vi "Top level_ Node FTP and STAT software.vi"() -> ()   [LabVIEW 2010]
uses:
  <vilib>/Utility/config.llb/NI_LVConfig.lvlib
  <vilib>/Utility/sysdir.llb/System Directory Type.ctl
  <vilib>/Utility/config.llb/Write Key (Boolean).vi
  FTP Credintials.ctl
panel:
  in  "Top level Tabs":enum32{"FTP Connection & Directories", "Page 2"}(tab)
  in  "Manual FTP":bool
  in  "Manual Archive":bool
  in  "ShutDown":bool
  in  "FTP Creds":T1 {"FTP Timeout (S)" min=0 max=10 step=1}
  in  "Archive Location 2":path caption="(Optional) External Directory To Archive *.RAT files"
  in  "Archive Location":path=path "C:/Archive" caption="Directory To Archive *.RAT files"
  in  "Rats Location":path=path "C:/Incoming" caption="Directory To Find *.RAT files"
  # "DIRECTORY SETUP"
  # "FTP SETUP"
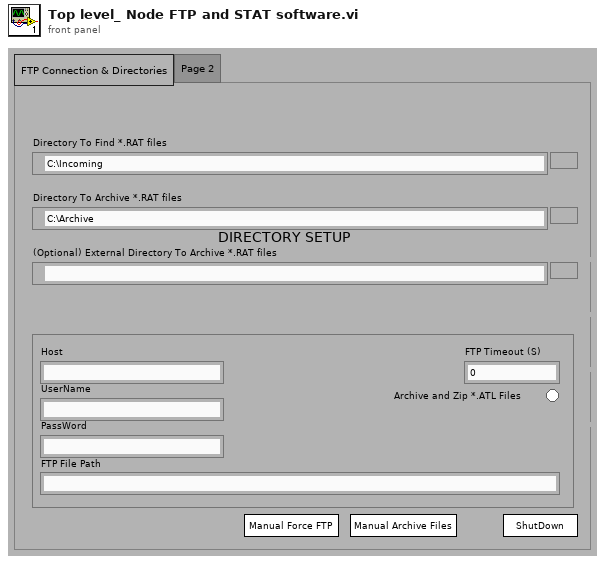
[diagram p1: front panel]
types:
  T1 = typedef "FTP Credintials.ctl" = cluster{"Host":string, "UserName":string, "PassWord":string, "FTP File Path":string, "FTP Timeout (S)":i32, "Use ATL":bool}
  T2 = typedef "System Directory Type.ctl" = i32
  T3 = cluster{"INI Section":string, "INI Key":string, "Use ATL":bool}
  T4 = cluster{"INI section (in)":string, "INI key (in)":string, "Value":string}
  T5 = typedef "NI_LVConfig.lvlib/Config Data RefNum.ctl" = refnum<k1>
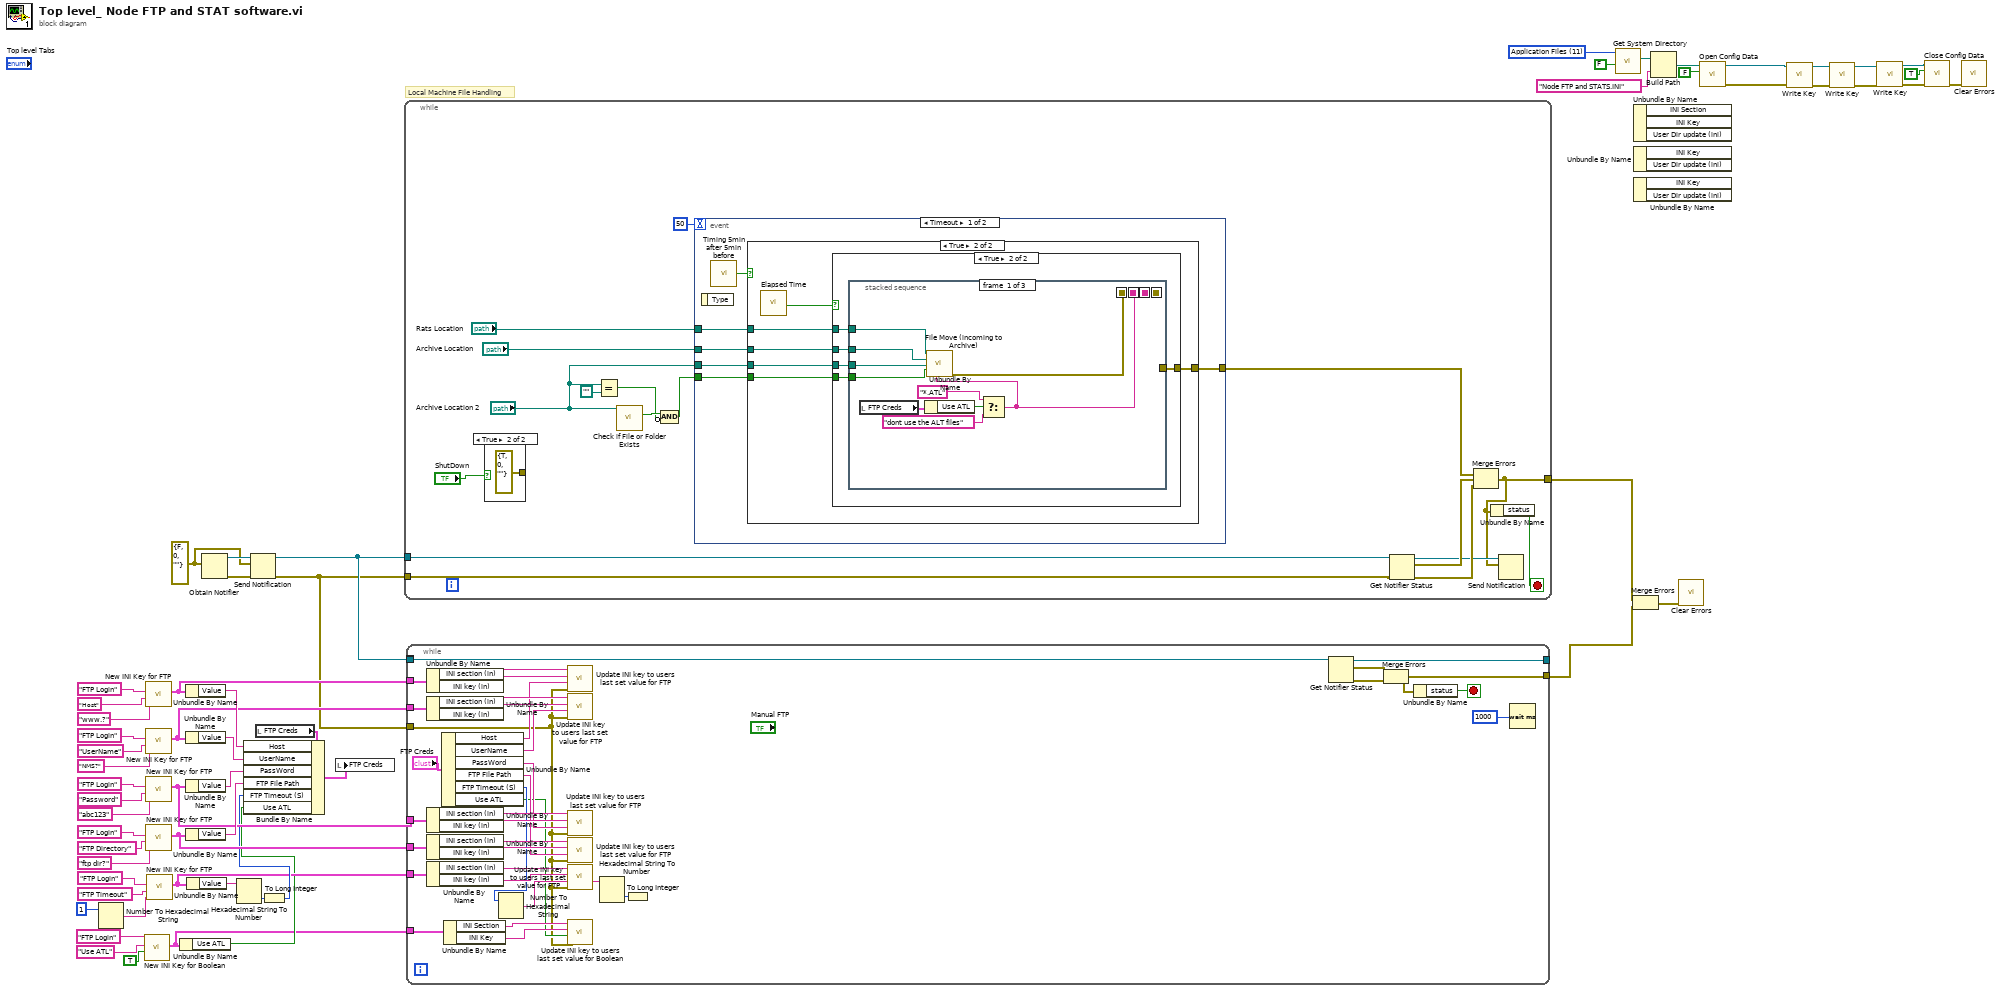
[diagram p0: block diagram]
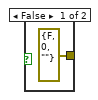
[diagram p2: hidden frame]
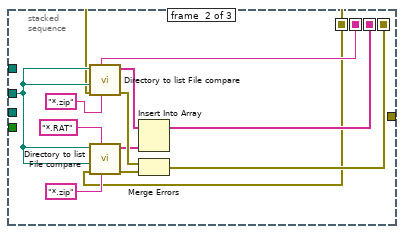
[diagram p5: hidden frame]
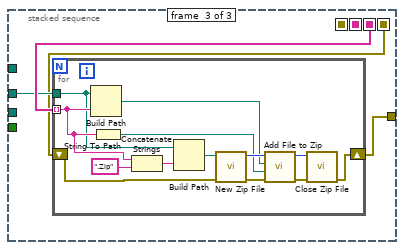
[diagram p6: hidden frame]
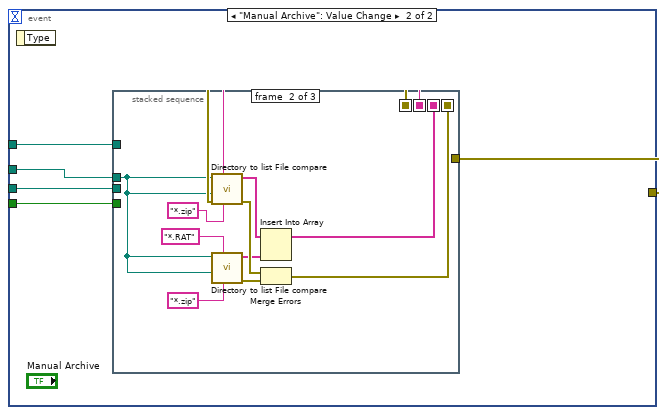
[diagram p7: hidden frame]
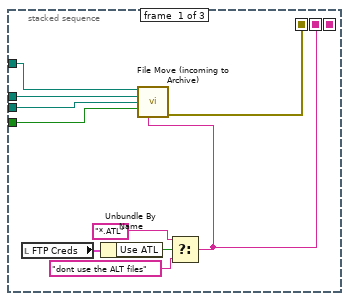
[diagram p8: hidden frame]
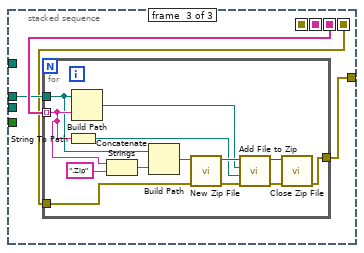
[diagram p9: hidden frame]
diagram:
  w15 = T2 11 items=["User Home"=0, "User Desktop"=1, "User Documents"=2, "User Application Data"=3, "User Preferences"=4, "User Temporary"=5, "Public Documents"=6, "Public Application Data"=7, "Public Preferences"=8, "Public Cache"=13, "System Core Libraries"=9, "System Installed Libraries"=10, "Application Files"=11, "Boot Volume Root"=12] ("system directory type")
  w23 = errorcluster {"status"=FALSE, "code"=0, "source"=""} ("error in (no error)")
  # "Local Machine File Handling"
  n1 = Number To Hexadecimal String(2:1) -> (0:w34:string)  [unwired: 1 in]
  n2 = call "New INI Key for Boolean.vi"("Use ATL"=TRUE, "INI key (in)"="Use ATL", "INI section (in)"="FTP Login") -> ("output cluster"=w25:T3)  [unwired: 8 in]
  n3 = call "New INI Key for FTP.vi"("Value"="www.?", "INI key (in)"="Host", "INI section (in)"="FTP Login") -> ("output cluster"=w43:T4)  [unwired: 7 in]
  n4 = call "New INI Key for FTP.vi"("Value"="NMS?", "INI key (in)"="UserName", "INI section (in)"="FTP Login") -> ("output cluster"=w42:T4)  [unwired: 7 in]
  n5 = call "New INI Key for FTP.vi"("Value"="abc123", "INI key (in)"="Password", "INI section (in)"="FTP Login") -> ("output cluster"=w41:T4)  [unwired: 7 in]
  n6 = call "New INI Key for FTP.vi"("Value"="ftp dir?", "INI key (in)"="FTP Directory", "INI section (in)"="FTP Login") -> ("output cluster"=w40:T4)  [unwired: 7 in]
  n7 = call "New INI Key for FTP.vi"("Value"=w34, "INI key (in)"="FTP Timeout", "INI section (in)"="FTP Login") -> ("output cluster"=w30:T4)  [unwired: 7 in]
  n8 = Unbundle By Name(w25) -> ("Use ATL"=w26:bool)
  n9 = Unbundle By Name(w43) -> ("Value"=w47:string)
  n10 = Unbundle By Name(w42) -> ("Value"=w46:string)
  n11 = Unbundle By Name(w41) -> ("Value"=w45:string)
  n12 = Unbundle By Name(w40) -> ("Value"=w44:string)
  n13 = Unbundle By Name(w30) -> ("Value"=w33:string)
  n14 = Obtain Notifier(notification data type=w23) -> (notifier out=w24:refnum<notifier>, error out=w22:errorcluster)  [unwired: 3 in, 1 out]
  n15 = Hexadecimal String To Number(string=w33) -> (number=w32:u32)  [unwired: 2 in, 1 out]
  n16 = Send Notification(notification=w23, notifier=w24, error in (no error)=w22) -> (notifier out=w21:refnum<notifier>, error out=w20:errorcluster)
  n17 = local read "FTP Creds"() -> (w38:T1)
  n18 = To Long Integer(number=w32) -> (32bit integer=w31:i32)
  n19 = Bundle By Name(cluster=w38, "Host"=w47, "UserName"=w46, "PassWord"=w45, "FTP File Path"=w44, "FTP Timeout (S)"=w31, "Use ATL"=w26) -> (w39:T1)
  n20 = local write "FTP Creds"(w39) -> ()
  n21 = while {
    tunnel: w21 -> [w71]
    tunnel: w20 -> [w69]
    tunnel: [w64] -> w19
    stop <- w67 stop-if-true
    n22 = case shown="True" "ShutDown" {
      tunnel: [errorcluster {"status"=FALSE, "code"=0, "source"=""} ("error in (no error)") errorcluster {"status"=TRUE, "code"=0, "source"=""} ("error in (no error)")] -> _
      frame False {
      }
      frame True {
      }
    }
    n23 = Equal?(x="Archive Location 2", y=path "") -> (x = y?=w74:bool)
    n24 = call <vilib>:"Check if File or Folder Exists.vi"("path"="Archive Location 2") -> ("file or folder exists?"=w75:bool)  [unwired: 8 in, 2 out]
    n25 = Compound Arithmetic op=AND(w75, invert w74) -> (w73:bool)
    n26 = event shown="[0] Timeout" {
      selector: _ -> [_ _]
      dyn-events: _ -> [_ _]
      timeout: 50 -> [_ _]
      tunnel: "Rats Location" -> [w84 w139]
      tunnel: "Archive Location" -> [w83 w138]
      tunnel: "Archive Location 2" -> [w82 w137]
      tunnel: w73 -> [w81 w136]
      tunnel: [w80 w135] -> w65
      event Timeout {
        n27 = event-data() -> ()  [unwired: 1 in, 1 out]
        n28 = call "Timing 5min after 5min before.vi"() -> ("Mid Hour"=w79:bool)  [unwired: 5 in]
        n29 = case shown="True" w79 {
          tunnel: w84 -> [_ w90]
          tunnel: w83 -> [_ w89]
          tunnel: w82 -> [_ w88]
          tunnel: w81 -> [_ w87]
          tunnel: [_ w86] -> w80
          frame False {
          }
          frame True {
            n30 = call "Elapsed Time"() -> ("Time has Elapsed"=w85:bool)  [unwired: 12 in, 7 out]
            n31 = case shown="True" w85 {
              tunnel: w90 -> [_ w95]
              tunnel: w89 -> [_ w94]
              tunnel: w88 -> [_ w93]
              tunnel: w87 -> [_ w92]
              tunnel: [_ w91] -> w86
              frame False {
              }
              frame True {
                n32 = stacked-sequence {
                  seq-local: [_ w107 _] -> [_ _ w121]
                  seq-local: [w101 _ _] -> [_ w113 _]
                  seq-local: [w100 _ _] -> [_ w106 _]
                  seq-local: [_ w110 _] -> [_ _ w119]
                  tunnel: w95 -> [w96 _ _]
                  tunnel: w94 -> [w97 w114 w120]
                  tunnel: w93 -> [w98 _ _]
                  tunnel: w92 -> [w99 _ _]
                  tunnel: [_ _ w118] -> w91
                  frame #0 {
                    n33 = local read "FTP Creds"() -> (w105:T1)
                    n34 = Unbundle By Name(w105) -> ("Use ATL"=w104:bool)
                    n35 = Select(t="*.ATL" ("pattern"), s=w104, f="dont use the ALT files" ("pattern")) -> (s? t:f=w101:string)
                    n36 = call "File Move (incoming to Archive).vi"("Rats Location"=w96, "Archive Location"=w97, "Archive Location 2"=w98, "Archive 2 valid path"=w99, "pattern"=w101) -> ("error IO"=w100:errorcluster)  [unwired: 10 in]
                  }
                  frame #1 {
                    n37 = call "Directory to list File compare.vi"("2nd File Type(s)(*.txt *.CSV)"="*.zip", "1st File Type(s)(*.txt *.CSV)"=w113, "error in (no error)"=w106, "2nd Directory (Zip)"=w114, "1st Directory (RATS)"=w114) -> ("error out"=w112:errorcluster, "Unmanaged Files"=w109:string[])  [unwired: 4 in, 1 out]
                    n38 = call "Directory to list File compare.vi"("2nd File Type(s)(*.txt *.CSV)"="*.zip", "1st File Type(s)(*.txt *.CSV)"="*.RAT" ("2nd File Type(s)(*.txt *.CSV)"), "error in (no error)"=w106, "2nd Directory (Zip)"=w114, "1st Directory (RATS)"=w114) -> ("error out"=w111:errorcluster, "Unmanaged Files"=w108:string[])  [unwired: 4 in, 1 out]
                    n39 = Insert Into Array(array=w109, new element=w108) -> (w107:string[])  [unwired: 1 in]
                    n40 = Merge Errors(w112, w111) -> (w110:errorcluster)
                  }
                  frame #2 {
                    n41 = for {
                      tunnel: w121 -> [w123] mode=indexing
                      tunnel: w120 -> [w122]
                      shift-right: [w128] -> w118
                      shift-left: w119 -> [w129]
                      n42 = Build Path(base path=w122, name or relative path=w123) -> (appended path=w126:path)
                      n43 = String To Path(string=w123) -> (path=w130:path)
                      n44 = Concatenate Strings(w123, ".Zip" ("name or relative path")) -> (w124:string)
                      n45 = Build Path(base path=w122, name or relative path=w124) -> (appended path=w127:path)
                      n46 = call <vilib>:"New Zip File.vi"("error in (no error)"=w129, "target"=w127) -> ("error out"=w131:errorcluster, "zip file out"=w134:i64)  [unwired: 3 in, 1 out]
                      n47 = call <vilib>:"Add File to Zip.vi"("error in (no error)"=w131, "destination path in zip"=w130, "source file path"=w126, "zip file in"=w134) -> ("error out"=w133:errorcluster, "zip file out"=w132:i64)  [unwired: 6 in]
                      n48 = call <vilib>:"Close Zip File.vi"("error in (no error)"=w133, "zip file in"=w132) -> ("error out"=w128:errorcluster)  [unwired: 5 in]
                    }
                  }
                }
              }
            }
          }
        }
      }
      event "Manual Archive": Value Change {
        n49 = event-data() -> ()  [unwired: 1 in, 1 out]
        n50 = stacked-sequence {
          seq-local: [_ w150 _] -> [_ _ w165]
          seq-local: [w141 _ _] -> [_ w156 _]
          seq-local: [w140 _ _] -> [_ w160 _]
          seq-local: [_ w153 _] -> [_ _ w163]
          tunnel: w139 -> [w142 _ _]
          tunnel: w138 -> [w143 w157 w164]
          tunnel: w137 -> [w144 _ _]
          tunnel: w136 -> [w145 _ _]
          tunnel: [_ _ w162] -> w135
          frame #0 {
            n51 = local read "FTP Creds"() -> (w149:T1)
            n52 = Unbundle By Name(w149) -> ("Use ATL"=w148:bool)
            n53 = Select(t="*.ATL" ("pattern"), s=w148, f="dont use the ALT files" ("pattern")) -> (s? t:f=w141:string)
            n54 = call "File Move (incoming to Archive).vi"("Rats Location"=w142, "Archive Location"=w143, "Archive Location 2"=w144, "Archive 2 valid path"=w145, "pattern"=w141) -> ("error IO"=w140:errorcluster)  [unwired: 10 in]
          }
          frame #1 {
            n55 = call "Directory to list File compare.vi"("2nd File Type(s)(*.txt *.CSV)"="*.zip", "1st File Type(s)(*.txt *.CSV)"=w156, "error in (no error)"=w160, "2nd Directory (Zip)"=w157, "1st Directory (RATS)"=w157) -> ("error out"=w155:errorcluster, "Unmanaged Files"=w152:string[])  [unwired: 4 in, 1 out]
            n56 = call "Directory to list File compare.vi"("2nd File Type(s)(*.txt *.CSV)"="*.zip", "1st File Type(s)(*.txt *.CSV)"="*.RAT" ("2nd File Type(s)(*.txt *.CSV)"), "2nd Directory (Zip)"=w157, "1st Directory (RATS)"=w157) -> ("error out"=w154:errorcluster, "Unmanaged Files"=w151:string[])  [unwired: 5 in, 1 out]
            n57 = Insert Into Array(array=w152, new element=w151) -> (w150:string[])  [unwired: 1 in]
            n58 = Merge Errors(w155, w154) -> (w153:errorcluster)
          }
          frame #2 {
            n59 = for {
              tunnel: w165 -> [w167] mode=indexing
              tunnel: w164 -> [w166]
              tunnel: w163 -> [w173]
              tunnel: [w172] -> w162
              n60 = String To Path(string=w167) -> (path=w174:path)
              n61 = Build Path(base path=w166, name or relative path=w167) -> (appended path=w170:path)
              n62 = Concatenate Strings(w167, ".Zip" ("name or relative path")) -> (w168:string)
              n63 = Build Path(base path=w166, name or relative path=w168) -> (appended path=w171:path)
              n64 = call <vilib>:"New Zip File.vi"("error in (no error)"=w173, "target"=w171) -> ("error out"=w175:errorcluster, "zip file out"=w178:i64)  [unwired: 3 in, 1 out]
              n65 = call <vilib>:"Add File to Zip.vi"("error in (no error)"=w175, "destination path in zip"=w174, "source file path"=w170, "zip file in"=w178) -> ("error out"=w177:errorcluster, "zip file out"=w176:i64)  [unwired: 6 in]
              n66 = call <vilib>:"Close Zip File.vi"("error in (no error)"=w177, "zip file in"=w176) -> ("error out"=w172:errorcluster)  [unwired: 5 in]
            }
          }
        }
      }
    }
    n67 = Get Notifier Status(notifier=w71, error in (no error)=w69) -> (notifier out=w66:refnum<notifier>, current notification=w70:errorcluster, error out=w68:errorcluster)  [unwired: 2 out]
    n68 = Merge Errors(w65, w70, w68) -> (w64:errorcluster)
    n69 = Unbundle By Name(w64) -> ("status"=w67:bool)
    n70 = Send Notification(notification=w64, notifier=w66) -> ()  [unwired: 1 in, 2 out]
  }
  n71 = while {
    tunnel: w43 -> [w214]
    tunnel: w42 -> [w205]
    tunnel: w41 -> [w204]
    tunnel: w40 -> [w198]
    tunnel: w30 -> [w197]
    tunnel: w25 -> [w189]
    tunnel: [w184] -> _
    tunnel: w21 -> [w184]
    tunnel: w20 -> [w185]
    tunnel: [w180] -> _
    tunnel: [w179] -> w18
    stop <- w181 stop-if-true
    n72 = Unbundle By Name(w214) -> ("INI section (in)"=w213:string, "INI key (in)"=w212:string)
    n73 = Unbundle By Name(w205) -> ("INI section (in)"=w210:string, "INI key (in)"=w211:string)
    n74 = Unbundle By Name(w204) -> ("INI section (in)"=w209:string, "INI key (in)"=w208:string)
    n75 = Unbundle By Name(w198) -> ("INI section (in)"=w206:string, "INI key (in)"=w207:string)
    n76 = Unbundle By Name(w197) -> ("INI section (in)"=w196:string, "INI key (in)"=w195:string)
    n77 = Unbundle By Name("FTP Creds") -> ("Host"=w202:string, "UserName"=w201:string, "PassWord"=w200:string, "FTP File Path"=w199:string, "FTP Timeout (S)"=w193:i32, "Use ATL"=w186:bool)
    n78 = Unbundle By Name(w189) -> ("INI Section"=w188:string, "INI Key"=w187:string)
    n79 = Number To Hexadecimal String(2:w193) -> (0:w194:string)  [unwired: 1 in]
    n80 = call "Update INI key to users last set value for FTP.vi"("error in (no error)"=w185, "Value in"=w202, "INI Key"=w212, "INI Section"=w213) -> ()  [unwired: 6 in, 2 out]
    n81 = call "Update INI key to users last set value for FTP.vi"("error in (no error)"=w185, "Value in"=w201, "INI Key"=w211, "INI Section"=w210) -> ()  [unwired: 6 in, 2 out]
    n82 = call "Update INI key to users last set value for FTP.vi"("error in (no error)"=w185, "Value in"=w200, "INI Key"=w208, "INI Section"=w209) -> ()  [unwired: 6 in, 2 out]
    n83 = call "Update INI key to users last set value for FTP.vi"("error in (no error)"=w185, "Value in"=w199, "INI Key"=w207, "INI Section"=w206) -> ()  [unwired: 6 in, 2 out]
    n84 = call "Update INI key to users last set value for FTP.vi"("error in (no error)"=w185, "Value in"=w194, "INI Key"=w195, "INI Section"=w196) -> ("Value out"=w191:string)  [unwired: 6 in, 1 out]
    n85 = call "Update INI key to users last set value for Boolean.vi"("error in (no error)"=w185, "TF for INI (in)"=w186, "INI Key"=w187, "INI Section"=w188) -> ()  [unwired: 6 in, 2 out]
    n86 = Hexadecimal String To Number(string=w191) -> (number=w192:u32)  [unwired: 2 in, 1 out]
    n87 = To Long Integer(number=w192) -> ()  [unwired: 1 out]
    n88 = Get Notifier Status(notifier=w184) -> (notifier out=w180:refnum<notifier>, current notification=w182:errorcluster, error out=w183:errorcluster)  [unwired: 1 in, 2 out]
    n89 = Merge Errors(w182, w183) -> (w179:errorcluster)
    n90 = Unbundle By Name(w179) -> ("status"=w181:bool)
    n91 = Wait (ms)(milliseconds to wait=u32 1000) -> ()  [unwired: 1 out]
  }
  n92 = call <vilib>:"Get System Directory.vi"("create directory if not found? (F)"=FALSE, "system directory type"=w15) -> ("system directory"=w14:path)  [unwired: 9 in]
  n93 = Merge Errors(w19, w18) -> (w17:errorcluster)
  n94 = Unbundle By Name() -> ()  [unwired: 1 in, 3 out]
  n95 = Unbundle By Name() -> ()  [unwired: 1 in, 2 out]
  n96 = Unbundle By Name() -> ()  [unwired: 1 in, 2 out]
  n97 = Build Path(base path=w14, name or relative path="Node FTP and STATS.INI") -> (appended path=w3:path)
  n98 = call <vilib>:"Clear Errors.vi"("error in (no error)"=w17) -> ()  [unwired: 6 in, 1 out]
  n99 = call <vilib>:"Open Config Data.vi"("create file if necessary (T)"=FALSE, "configuration file path"=w3) -> ("error out"=w4:errorcluster, "refnum"=w5:T5)  [unwired: 7 in, 1 out]
  n100 = call-poly <vilib>:"Write Key.vi"("error in (no error)"=w4, "refnum"=w5) -> ("error out"=w7:errorcluster, "refnum out"=w6:T5)  [unwired: 7 in, 1 out]
  n101 = call-poly <vilib>:"Write Key.vi"("error in (no error)"=w7, "refnum"=w6) -> ("error out"=w9:errorcluster, "refnum out"=w8:T5)  [unwired: 7 in, 1 out]
  n102 = call-poly <vilib>:"Write Key.vi"("error in (no error)"=w9, "refnum"=w8) -> ("error out"=w12:errorcluster, "refnum out"=w10:T5)  [unwired: 7 in, 1 out]
  n103 = call <vilib>:"Close Config Data.vi"("error in (no error)"=w12, "write file if changed (T)"=TRUE, "refnum"=w10) -> ("error out"=w2:errorcluster)  [unwired: 7 in, 1 out]
  n104 = call <vilib>:"Clear Errors.vi"("error in (no error)"=w2) -> ()  [unwired: 6 in, 1 out]
